vi "cnc-product.vi"(2 "speed in":i32(listbox), 3 "Products in":u16) -> (1 "Products out":u16)   [LabVIEW 2026]
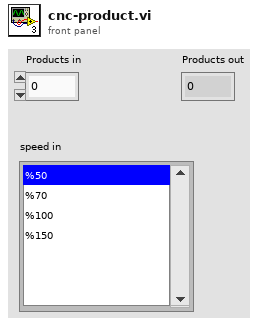
[diagram p1: front panel]
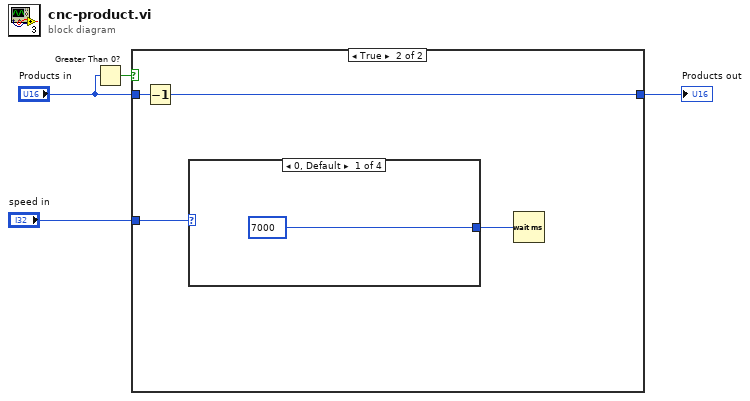
[diagram p0: block diagram]
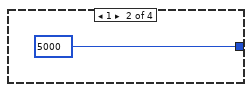
[diagram p3: hidden frame]
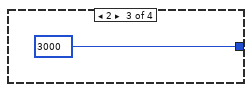
[diagram p4: hidden frame]
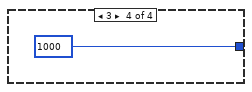
[diagram p5: hidden frame]
diagram:
  n1 = Greater Than 0?(x="Products in") -> (x > 0?=w4:bool)
  n2 = case shown="True" w4 {
    tunnel: "Products in" -> [w5 w9]
    tunnel: [w5 w8] -> w2
    tunnel: "speed in" -> [_ w6]
    frame False {
    }
    frame True {
      n3 = Decrement(x=w9) -> (x-1=w8:u16)
      n4 = case shown="0, Default" w6 {
        tunnel: [u16 7000 ("Products in") u16 5000 ("Products in") u16 3000 ("Products in") u16 1000 ("Products in")] -> w7
        frame 0, Default {
        }
        frame 1 {
        }
        frame 2 {
        }
        frame 3 {
        }
      }
      n5 = Wait (ms)(milliseconds to wait=w7) -> ()  [unwired: 1 out]
    }
  }
  "Products out" <- w2
